vi "testing_readMeasurementsSingles.vi"() -> ()   [LabVIEW 2015, in "Tausand AB1000.lvlib"]
uses:
  <instrlib>/Tausand AB1000/Tausand AB1000.lvlib
  <instrlib>/Tausand AB1000/Public/Controls/deviceTypeRing.ctl
  <vilib>/Analysis/NI_AALBase.lvlib
panel:
  out "num reads":i32
  in  "intervals":i32=20
  out "stddev (s)":dbl format="%0.4f"
  out "min (s)":dbl format="%0.4f"
  out "max (s)":dbl format="%0.4f"
  out "mean (s)":dbl format="%0.4f"
  out "reading timer histogram":T1(graph)
  in  "stop":bool
  out "last reading timer (s)":dbl format="%0.4f"
  out "error out":errorcluster
  in  "VISA resource name":refnum<visa-resource-name>
  in  "error in (no error)":errorcluster
  out "checksum ok?":bool
  out "read time":timestamp
  out "labels":string[](array[string])
  out "values":u32[](array[numeric])
  in  "read timeout (500 ms)":u32=500
  in  "device type":T2 items=["any"=0, "AB1002"=1002, "AB1004"=1004, "AB1502"=1502, "AB1504"=1504, "AB2002"=2002, "AB2004"=2004, "AB2502"=2502, "AB2504"=2504]
  # "TEST of: 'Read singles counters.vi'"
  # "Reading timer statistics"
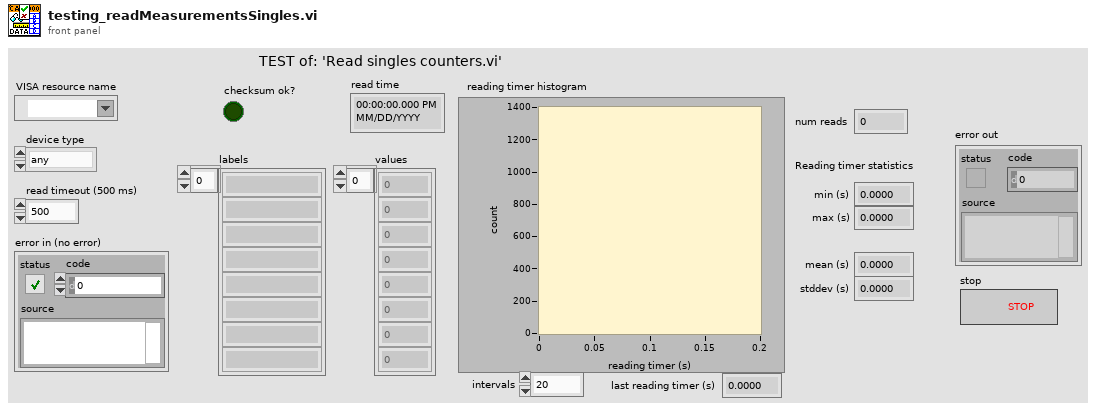
[diagram p1: front panel]
types:
  T1 = cluster{"X Values":dbl[], "Histogram: h(x)":i32[]}
  T2 = typedef "Tausand AB1000.lvlib/deviceTypeRing.ctl" = u16
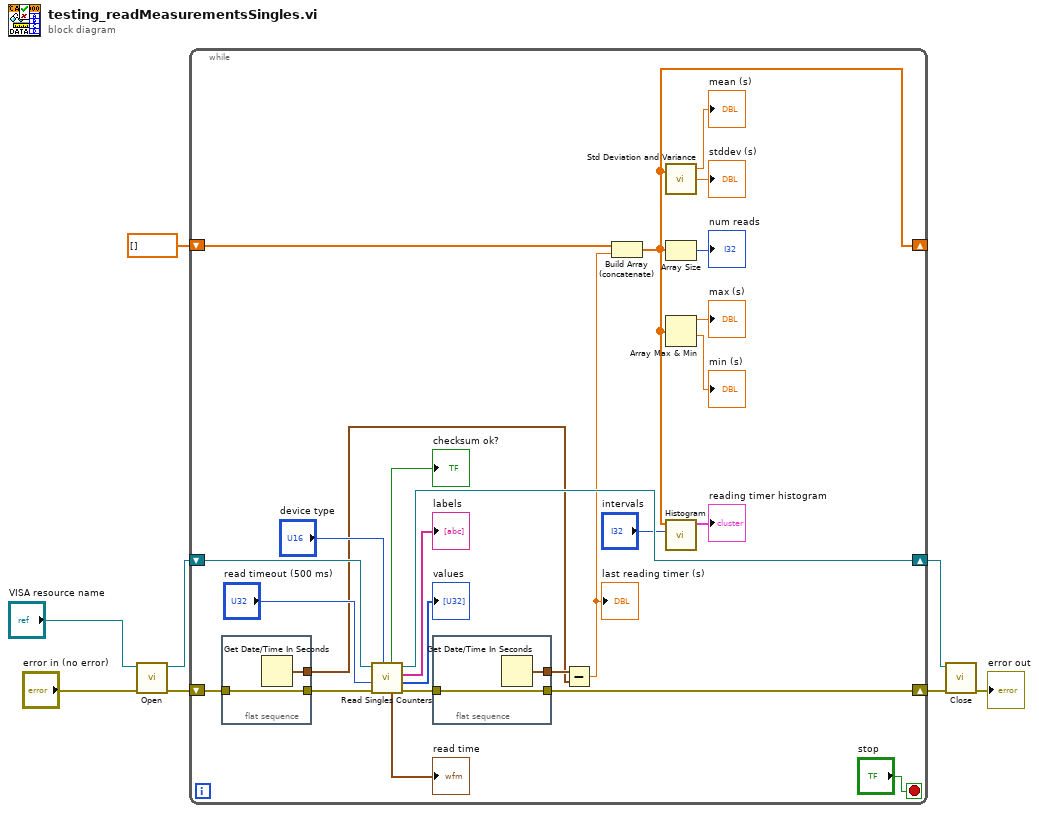
[diagram p0: block diagram]
diagram:
  n1 = call <instrlib>:"Open.vi"("error in (no error)"="error in (no error)", "VISA resource name"="VISA resource name") -> ("error out"=w3:errorcluster, "VISA resource name out"=w8:refnum<visa-resource-name>)  [unwired: 8 in]
  n2 = while {
    shift-right: [w32] -> w7
    shift-left: w8 -> [w33]
    shift-right: [w22] -> w2
    shift-left: w3 -> [w24]
    shift-right: [w10] -> _
    shift-left: dbl[] [] -> [w17]
    stop <- "stop" stop-if-true
    n3 = flat-sequence {
      tunnel: [w37] -> w25
      tunnel: w24 -> [w37]
      tunnel: [w36] -> w20
      frame #0 {
        n4 = Get Date/Time In Seconds() -> (seconds since 1Jan1904=w36:timestamp)
      }
    }
    n5 = call <instrlib>:"Read Singles Counters.vi"("device type"="device type", "error in (no error)"=w25, "read timeout (500 ms)"="read timeout (500 ms)", "VISA Refnum in"=w33) -> ("error out"=w23:errorcluster, "values"=→"values":u32[], "labels"=→"labels":string[], "VISA Refnum out"=w32:refnum<visa-resource-name>, "read time"=→"read time":timestamp, "checksum ok?"=→"checksum ok?":bool)  [unwired: 2 in]
    n6 = flat-sequence {
      tunnel: [w35] -> w22
      tunnel: w23 -> [w35]
      tunnel: [w34] -> w21
      frame #0 {
        n7 = Get Date/Time In Seconds() -> (seconds since 1Jan1904=w34:timestamp)
      }
    }
    n8 = Subtract(x=w21, y=w20) -> (x-y=w18:dbl)
    "last reading timer (s)" <- w18
    n9 = Build Array (concatenate)(w17, w18) -> (w10:dbl[])
    n10 = call <vilib>:"Std Deviation and Variance.vi"("X"=w10) -> ("mean"=→"mean (s)":dbl, "standard deviation"=→"stddev (s)":dbl)  [unwired: 1 in, 1 out]
    n11 = Array Size(array=w10) -> (size(s)=→"num reads":i32)
    n12 = Array Max & Min(array=w10) -> (max value=→"max (s)":dbl, min value=→"min (s)":dbl)  [unwired: 2 out]
    n13 = call <vilib>:"Histogram.vi"("intervals"="intervals", "X"=w10) -> ("Histogram Graph"=→"reading timer histogram":T1)  [unwired: 6 in, 3 out]
  }
  n14 = call <instrlib>:"Close.vi"("error in (no error)"=w2, "VISA resource name"=w7) -> ("error out"=→"error out":errorcluster)  [unwired: 9 in]
